vi "ReadConfig.vi"(0 "reference in":refnum<class "Stand.lvclass">, 11 "error in (no error)":errorcluster) -> (4 "reference out":refnum<class "Stand.lvclass">, 15 "error out":errorcluster)   [LabVIEW 2019, in "Stand.lvclass"]
uses:
  Stand.lvclass
  C:/Users/ANENKOV_V1/Desktop/src/Device_class/Device.lvclass
  C:/Users/ANENKOV_V1/Desktop/src/Proccess_class/Proccess.lvclass
  Proccess_class/Proccess.lvclass/Proccess.ctl
  Device_class/Device.lvclass/Device.ctl
  Stand.lvclass/Stand.ctl
  32b4956d-1d2c-430c-854c-873c41fce1cb.vi
  <vilib>/Utility/error.llb/Clear Errors.vi
  ConfigInterface_class/ConfigInterface.lvclass
  Proccess_class/Proccess.lvclass
  Device_class/Device.lvclass
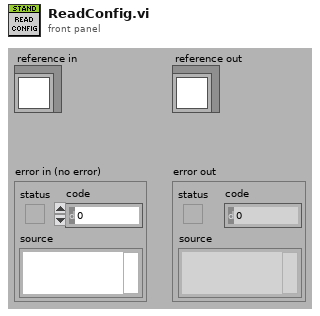
[diagram p1: front panel]
types:
  T1 = typedef "Setting Stand.ctl" = cluster{"Pressure Source":T2, "dt pressure down ms":i32, "dP pressure down MPa":dbl, "Haskel":T3, "Pump":T3, "Accuracy [%]":dbl, "Accuracy max [MPa]":dbl, "Accuracy min [MPa]":dbl, "BackPressurVoltage [V]":dbl}
  T2 = typedef "Pressure Source.ctl" = enum16{"Internal", "Modbus", "UDP"}
  T3 = typedef "Setting Pressure PI.ctl" = cluster{"A [MPa/V]":dbl, "P0 [MPa]":dbl}
  T4 = typedef "Proccess.lvclass/TAGs.ctl" = cluster{"TAG":string, "PTAG":string, "DESC":string}
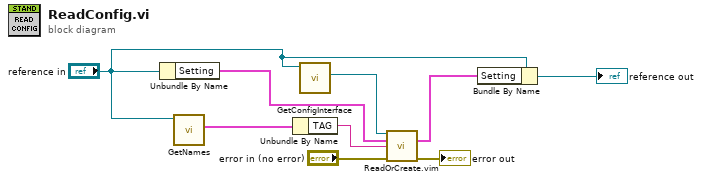
[diagram p0: block diagram]
diagram:
  n1 = Unbundle By Name("reference in") -> ("Setting"=w8:T1)
  n2 = call "GetNames.vi"("Proccess in"="reference in") -> ("Tags"=w6:T4)  [unwired: 10 in]
  n3 = Unbundle By Name(w6) -> ("TAG"=w1:string)
  n4 = call "GetConfigInterface.vi"("Device in"="reference in") -> ("ConfigInterface"=w9:refnum<class "ConfigInterface.lvclass">)  [unwired: 10 in]
  n5 = call "ReadOrCreate.vim"("reference in"=w9, "Type and Defaults"=w8, "Name"=w1, "error in (no error)"="error in (no error)") -> ("Data"=w3:T1, "error out"=→"error out":errorcluster)  [unwired: 7 in, 3 out]
  n6 = Bundle By Name(cluster="reference in", "Setting"=w3) -> (→"reference out":refnum<class "Stand.lvclass">)
